vi "Insert Key Value Pair (Single Numeric).vi"(7 "key":string, 8 "error in (no error)":errorcluster, 10 "value":dbl, 11 "JSON Object in":refnum<class "JSON Helper.lvclass">) -> (0 "error out":errorcluster, 1 "replaced":bool, 3 "JSON Object out":refnum<class "JSON Helper.lvclass">)   [LabVIEW 2016, in "JSON Helper.lvclass"]
uses:
  JSON Helper/JSON Helper.lvclass
  JSON Numeric/New JSON Numeric.vi
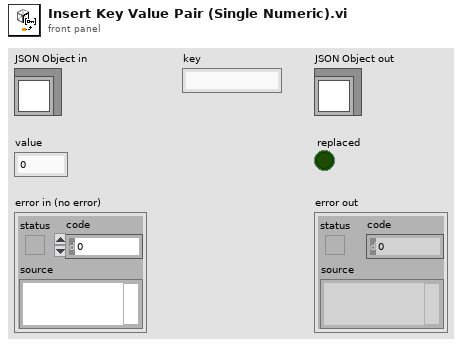
[diagram p1: front panel]
types:
  T1 = typedef "JSON Helper.lvclass/JSON Types.ctl" = enum16{"String", "Numeric", "Boolean", "NULL", "Object", "Array"}
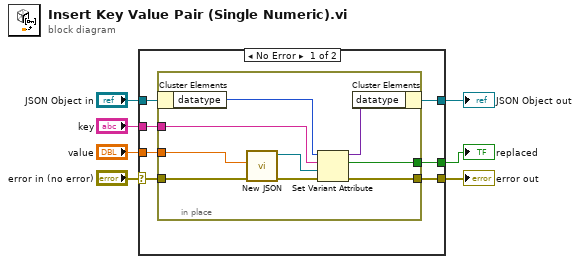
[diagram p0: block diagram]
diagram:
  n1 = case shown="No Error" "error in (no error)" {
    selector: "error in (no error)" -> [w10 w25]
    tunnel: [w9 w25] -> w6
    tunnel: [w13 w24] -> w4
    tunnel: "JSON Object in" -> [w14 w24]
    tunnel: "key" -> [w12 _]
    tunnel: "value" -> [w11 _]
    tunnel: [w8 _] -> w1
    frame No Error {
      n2 = in-place {
        in-place-border: w12 -> [w22]
        in-place-border: w11 -> [w17]
        in-place-border: w10 -> [w19]
        in-place-border: [w20] -> w9
        in-place-border: [w15] -> w8
        n3 = in-place-cluster #1(w14) -> ("datatype"=w23:T1)
        n4 = call-poly "New JSON.vi"("error in (no error)"=w19, "value"=w17) -> ("error out"=w18:errorcluster, "JSON String out"=w16:refnum<class "JSON Helper.lvclass">)  [unwired: 8 in]
        n5 = Set Variant Attribute(Variant=w23, name=w22, value=w16, error in=w18) -> (Variant out=w21:variant, replaced=w15:bool, error out=w20:errorcluster)
        n6 = in-place-cluster #1("datatype"=w21) -> (w13:refnum<class "JSON Helper.lvclass">)
      }
    }
    frame Error {
    }
  }
  "error out" <- w6
  "JSON Object out" <- w4
  "replaced" <- w1
